vi "UpdateCurserIdx(SubVI).vi"(8 "error in (no error)":errorcluster, 11 "WaveformGraph in":refnum<vi>) -> (0 "error out":errorcluster)   [LabVIEW 2020]
uses:
  GlobalVariables.vi
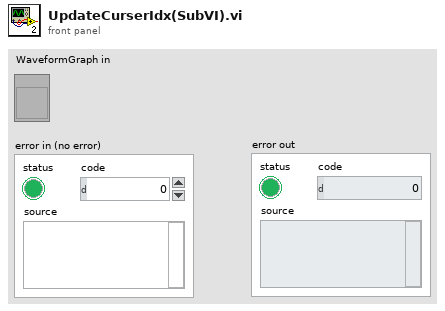
[diagram p1: front panel]
types:
  T1 = typedef "LVCursorListTypeDef.ctl" = cluster{"Name":string, "Color":u32, "Style":u8, "Point Style":u8, "Name Visible":bool, "Allow Drag":bool, "Cursor Mode":u32, "Plot":i32, "Index":i32, "Position":cluster{"X":dbl, "Y":dbl}, "X Scale":u32, "Y Scale":u32, "Watch Plots":i32[], "Watch All Plots":bool, "Plot Area":i32, "Label Offset":cluster{"X":dbl, "Y":dbl}}[]
  T2 = cluster{"Name":string, "Color":u32, "Style":u8, "Point Style":u8, "Name Visible":bool, "Allow Drag":bool, "Cursor Mode":u32, "Plot":i32, "Index":i32, "Position":cluster{"X":dbl, "Y":dbl}, "X Scale":u32, "Y Scale":u32, "Watch Plots":i32[], "Watch All Plots":bool, "Plot Area":i32, "Label Offset":cluster{"X":dbl, "Y":dbl}}
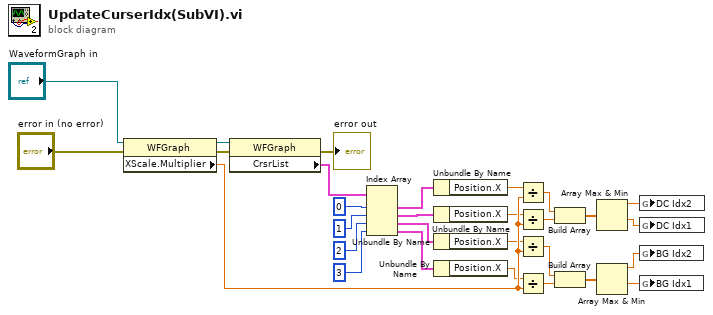
[diagram p0: block diagram]
diagram:
  n1 = property class="WFGraph"(reference="WaveformGraph in", error in="error in (no error)") -> (reference out=w11:refnum<vi>, error out=w12:errorcluster, "XScale.Multiplier"=w26:dbl)
  n2 = property class="WFGraph"(reference=w11, error in=w12) -> (error out=→"error out":errorcluster, "CrsrList"=w28:T1)  [unwired: 1 out]
  n3 = Index Array(array=w28, index #1=0 ("index"), index #2=1 ("index"), index #3=2 ("index"), index #4=3 ("index")) -> (element #1=w18:T2, element #2=w19:T2, element #3=w20:T2, element #4=w21:T2)
  n4 = Unbundle By Name(w18) -> ("Position.X"=w22:dbl)
  n5 = Unbundle By Name(w19) -> ("Position.X"=w23:dbl)
  n6 = Unbundle By Name(w20) -> ("Position.X"=w24:dbl)
  n7 = Unbundle By Name(w21) -> ("Position.X"=w25:dbl)
  n8 = Divide(x=w22, y=w26) -> (x/y=w10:dbl)
  n9 = Divide(x=w23, y=w26) -> (x/y=w9:dbl)
  n10 = Divide(x=w24, y=w26) -> (x/y=w4:dbl)
  n11 = Divide(x=w25, y=w26) -> (x/y=w3:dbl)
  n12 = Build Array(w10, w9) -> (w8:dbl[])
  n13 = Build Array(w4, w3) -> (w5:dbl[])
  n14 = Array Max & Min(array=w8) -> (max value=w7:dbl, min value=w6:dbl)  [unwired: 2 out]
  n15 = Array Max & Min(array=w5) -> (max value=w2:dbl, min value=w1:dbl)  [unwired: 2 out]
  n16 = global write "GlobalVariables.vi" "DC Idx2"(w7) -> ()
  n17 = global write "GlobalVariables.vi" "DC Idx1"(w6) -> ()
  n18 = global write "GlobalVariables.vi" "BG Idx2"(w2) -> ()
  n19 = global write "GlobalVariables.vi" "BG Idx1"(w1) -> ()
